vi "Drop Message Core.vi"(11 "Pick up Item Msg in":refnum<class "Pick up Item Msg.lvclass">) -> ()   [LabVIEW 2023, in "Customer.lvlib" / "Pick up Item Msg.lvclass"]
doc: "(<B>Filename</B>: Actor Framework.lvlib:Message.lvclass:Drop Message Core.vi)\n\nDefines what a message does if it is in the message queue when the queue is released. At this point, the actor has shut down, so it will never process the message.\n\nBy default, this method does nothing. A child class may override it to define behavior. National Instruments provides the Reply Msg class to override this method. This class releases its internal queue, which causes any caller of the Send Message and Wait For Response method to stop waiting and return an error."
uses:
  Pick up Item Msg.lvclass
  Pick up Item Msg.lvclass/Pick up Item Msg.ctl
  <vilib>/ActorFramework/Message/Message.lvclass
  Beverages/Beverage/Beverage.lvclass
panel:
  out "error out":errorcluster
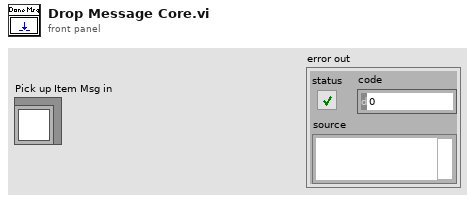
[diagram p1: front panel]
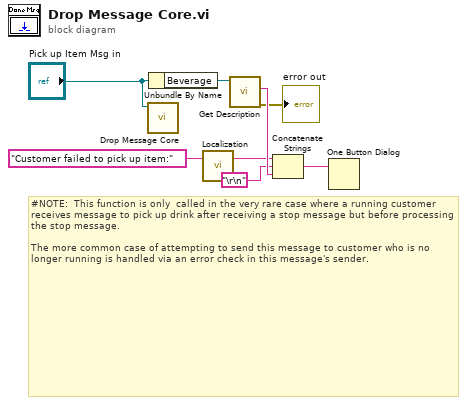
[diagram p0: block diagram]
diagram:
  # "#NOTE:  This function is only  called in the very rare case where a running customer receives message to pick up drink after receiving a stop message but before processing the stop message.\n\nThe more common case of attempting to send this message to customer who is no longer running is handled via an error check in this message's sender."
  n1 = call-parent "Drop Message Core.vi"("Message in"="Pick up Item Msg in") -> ()  [unwired: 11 in]
  n2 = Unbundle By Name("Pick up Item Msg in") -> ("Beverage"=w7:refnum<class "Beverage.lvclass">)
  n3 = call "Localization.vi"("untranslated"="Customer failed to pick up item:" ("Status")) -> ("translated"=w2:string)  [unwired: 2 in]
  n4 = call "Get Description.vi"("Beverage in"=w7) -> ("error out"=→"error out":errorcluster, "Description"=w5:string)  [unwired: 8 in, 1 out]
  n5 = Concatenate Strings(w2, "\r\n", w5) -> (w6:string)
  n6 = One Button Dialog(message=w6) -> ()  [unwired: 1 in, 1 out]
